vi "19- Arduino analog sensor data on graph.vi"() -> ()   [LabVIEW 2019]
uses:
  <vilib>/MakerHub/LINX/Public/Peripherals/Analog/Analog Read 1 Chan.vi
  <vilib>/MakerHub/LINX/Public/Peripherals/Analog/Analog Read N Chans.vi
  <vilib>/MakerHub/LINX/Private/Local IO/LinxAnalogRead.vi
  <vilib>/MakerHub/LINX/Public/Utilities/Check Channel.vi
  <vilib>/MakerHub/LINX/Public/Utilities/Open Serial.vi
  <vilib>/MakerHub/LINX/Private/Utilties/Generate Error.vi
  <vilib>/MakerHub/LINX/LMH-LINX.lvlib
panel:
  out "Waveform Graph":dbl[](graph)
  in  "stop":bool
  in  "Analog Channel":u8
  in  "Serial Port":refnum<visa-resource-name>="N/A"
  # "Arduino analog sensor data on waveform graph"
  # "Arduino configuration"
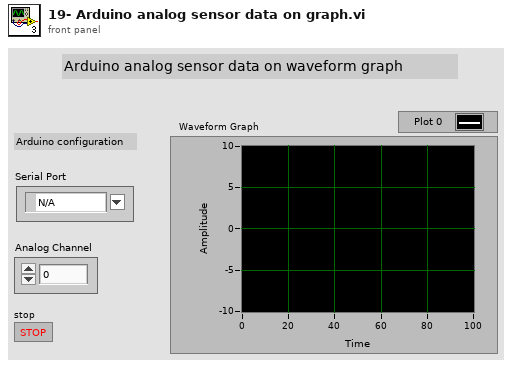
[diagram p1: front panel]
types:
  T1 = typedef "LMH-LINX.lvlib/LINX Ref.ctl" = cluster{"IO":T2, "Interface":T3, "LINX Device Config":T4}
  T2 = typedef "LMH-LINX.lvlib/Platform.ctl" = enum16{"Remote", "Local"}
  T3 = typedef "LMH-LINX.lvlib/Interface.ctl" = enum16{"Serial", "TCP"}
  T4 = typedef "LMH-LINX.lvlib/Device.lvlib/LINX Device Config.ctl" = cluster{"Interface":T3, "COM Port":refnum<visa-resource-name>, "TCP Configuration":T5, "Device Family":u8, "Device ID":u8, "Device Name":string, "TCP Ref":refnum<k5>, "Channels":T6}
  T5 = typedef "LMH-LINX.lvlib/Device.lvlib/TCP Config.ctl" = cluster{"IP Address":string, "Port":u16}
  T6 = typedef "LMH-LINX.lvlib/Channels.ctl" = cluster{"DI":u8[], "DO":u8[], "AI":u8[], "AO":u8[], "PWM":u8[], "QE":u8[], "UART":u8[], "I2C 2":u8[], "SPI":u8[], "CAN":u8[], "Servo":u8[], "AI Ref (V)":dbl, "AI Resolution (Bits)":u8, "AO Ref (V)":dbl, "AO Resolution (Bits)":u8}
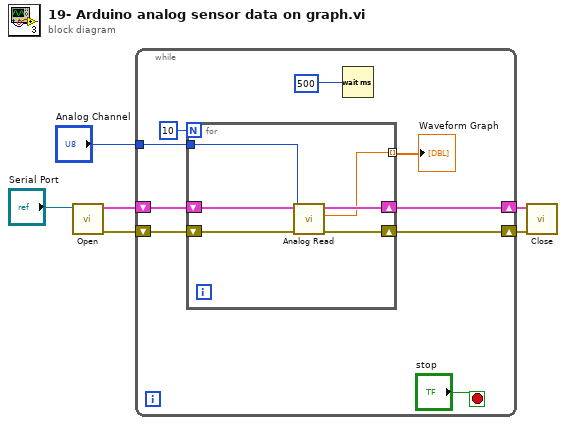
[diagram p0: block diagram]
diagram:
  n1 = call-poly <vilib>:"Open.vi"("Serial Port"="Serial Port") -> ("Error Out"=w6:errorcluster, "LINX Resource"=w3:T1)  [unwired: 8 in, 1 out]
  n2 = while {
    tunnel: "Analog Channel" -> [w11]
    shift-right: [w14] -> w5
    shift-left: w6 -> [w15]
    shift-right: [w12] -> w2
    shift-left: w3 -> [w13]
    stop <- "stop" stop-if-true
    n3 = for {
      N: 10 -> [_]
      tunnel: w11 -> [w17]
      shift-right: [w20] -> w14
      shift-left: w15 -> [w21]
      shift-right: [w18] -> w12
      shift-left: w13 -> [w19]
      tunnel: [w16] -> w8 mode=indexing
      n4 = call-poly <vilib>:"Analog Read.vi"("Error In"=w21, "Analog Channel"=w17, "LINX Resource"=w19) -> ("Error Out"=w20:errorcluster, "Voltage"=w16:dbl, "LINX Resource"=w18:T1)  [unwired: 5 in, 1 out]
    }
    "Waveform Graph" <- w8
    n5 = Wait (ms)(milliseconds to wait=u32 500 ("millisecond timer value")) -> ()  [unwired: 1 out]
  }
  n6 = call <vilib>:"Close.vi"("Error In"=w5, "LINX Resource"=w2) -> ()  [unwired: 9 in, 1 out]
